vi "saturation curves.vi"(10 "fluid name":u16, 11 "Units in":string(combo)="IP") -> (1 "XY Graph 3":cluster{dbl[], dbl[]}(graph), 2 "pT":cluster{dbl[], dbl[]}, 3 "Units out":string, 4 "Ts Diagram":cluster{dbl[], dbl[]}[](graph), 5 "Ts Sat Curve":cluster{dbl[], dbl[]}, 6 "ph Diagram":cluster{dbl[], dbl[]}[](graph), 7 "ph Sat Curve":cluster{dbl[], dbl[]})   [LabVIEW 2017]
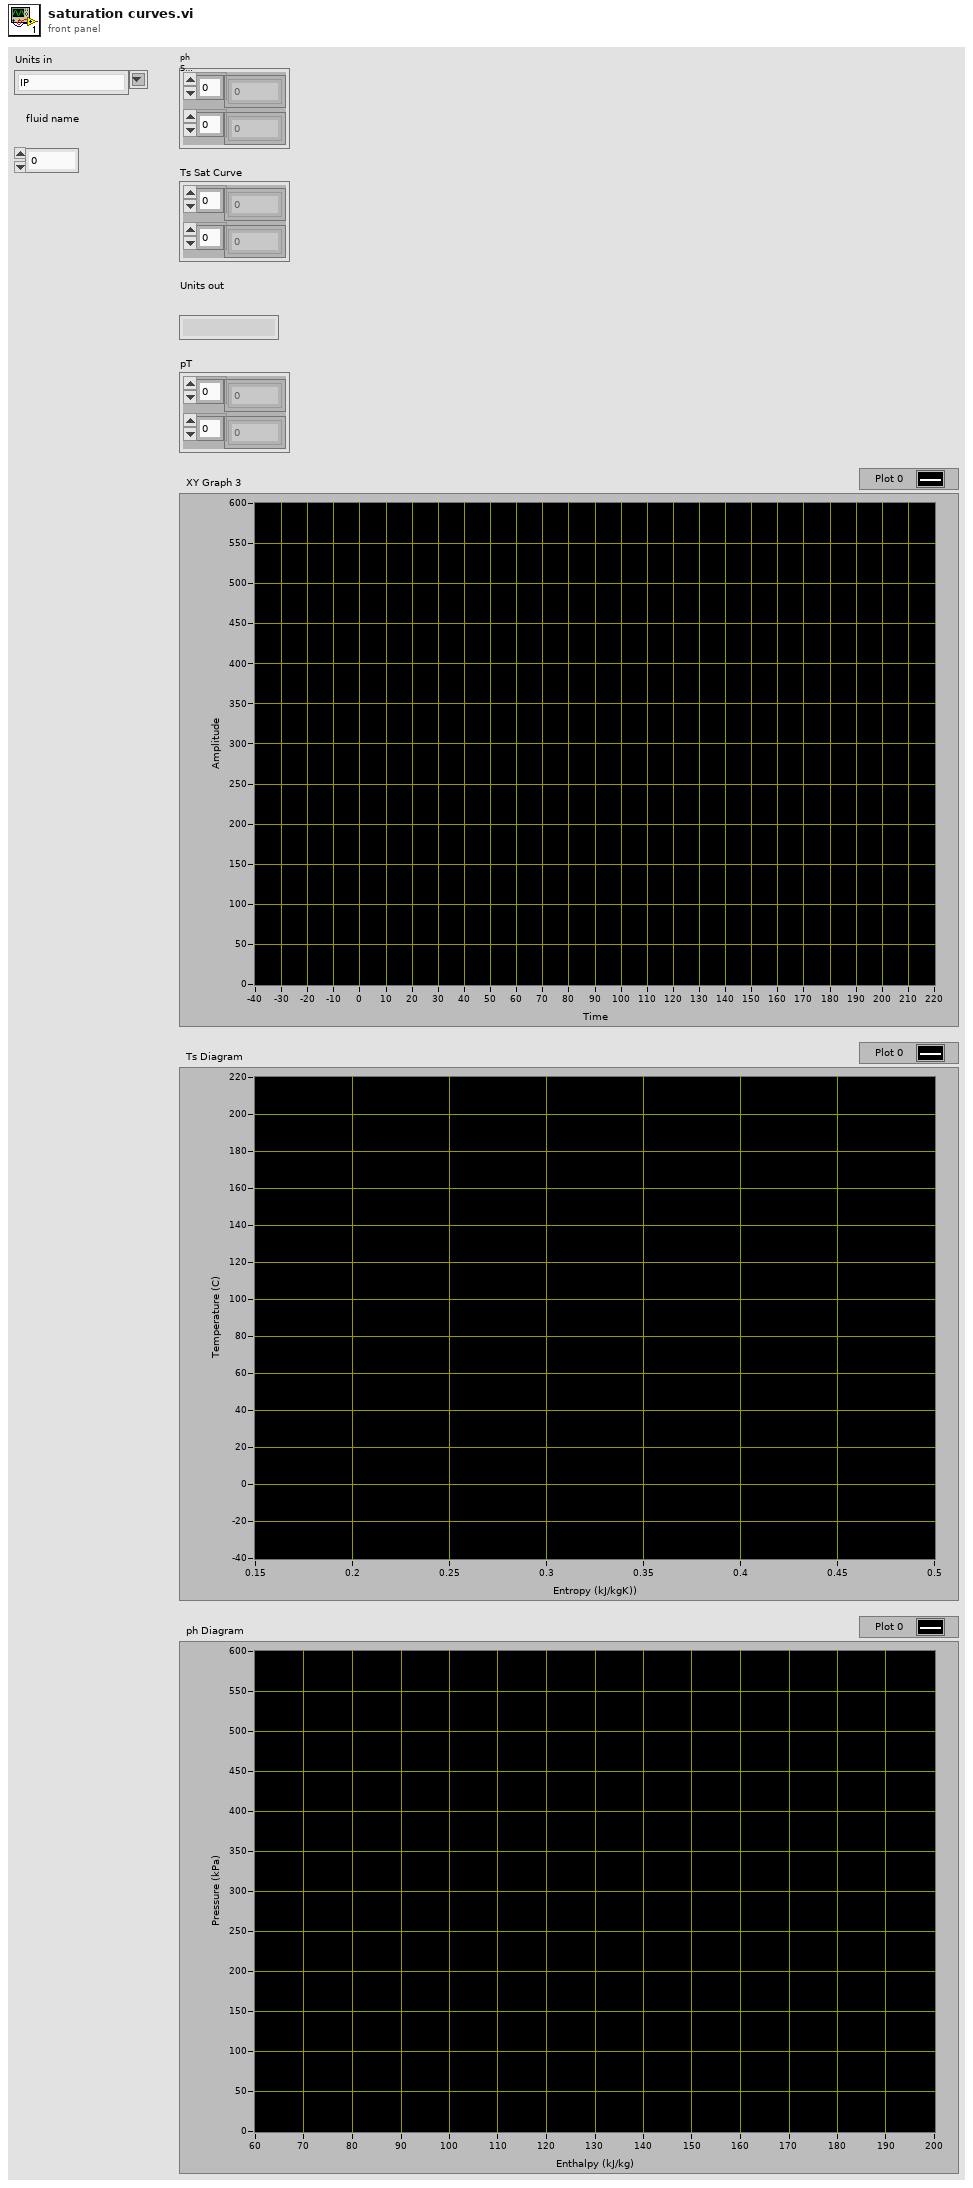
[diagram p1: front panel]
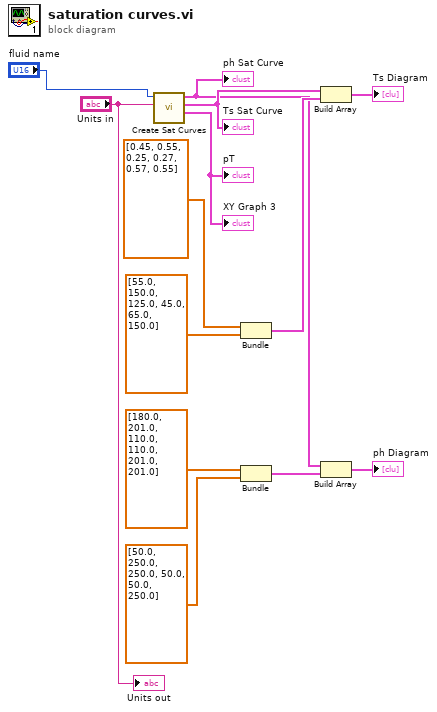
[diagram p0: block diagram]
diagram:
  n1 = call "Create Sat Curves.vi"("units"="Units in", "fluid name"="fluid name") -> ("pT"=→"pT" →"XY Graph 3":cluster{dbl[], dbl[]}, "Ts"=w5:cluster{dbl[], dbl[]}, "ph"=w2:cluster{dbl[], dbl[]})  [unwired: 7 in]
  "ph Sat Curve" <- w2
  "Ts Sat Curve" <- w5
  n2 = Bundle(dbl[] [0.45, 0.55, 0.25, 0.27, 0.57, 0.55], dbl[] [55.0, 150.0, 125.0, 45.0, 65.0, 150.0]) -> (w6:cluster{dbl[], dbl[]})  [unwired: 1 in]
  n3 = Bundle(dbl[] [180.0, 201.0, 110.0, 110.0, 201.0, 201.0], dbl[] [50.0, 250.0, 250.0, 50.0, 50.0, 250.0]) -> (w3:cluster{dbl[], dbl[]})  [unwired: 1 in]
  n4 = Build Array(w5, w6) -> (→"Ts Diagram":cluster{dbl[], dbl[]}[])
  n5 = Build Array(w2, w3) -> (→"ph Diagram":cluster{dbl[], dbl[]}[])
  "Units out" <- "Units in"
